vi "GeneralConfigMain.vi"(6 "NameSpace(Config)":string="Config", 8 "RIOfileName":string, 9 "Stop_Notifier":refnum<notifier>, 10 "IP_Notifier":refnum<notifier>, 11 "BasePath":path) -> ()   [LabVIEW 2016]
panel:
  in  "ViewCfgOnBot":bool
  in  "ULConfigtoRIO":bool
  in  "ConfigSaves":i32(listbox)=9
  in  "ConfigName":string
  in  "DeleteConfig":bool
  in  "LoadConfig":bool
  in  "SaveConfig":bool
  in  "Tab Control":enum32{"Page 1", "Page 2"}(tab)
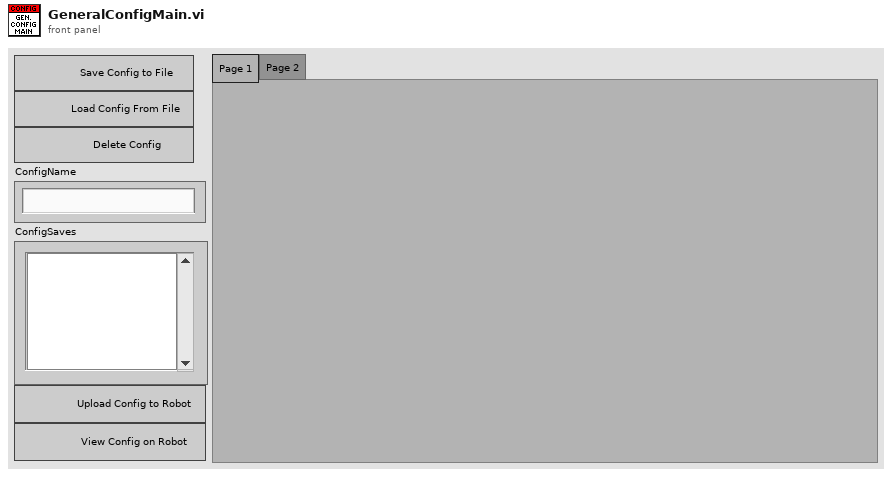
[diagram p1: front panel]
types:
  T1 = cluster{"ViewCfgOnBot":refnum<vi>, "ULConfigtoRIO":refnum<vi>, "ConfigSaves":refnum<vi>, "ConfigName":refnum<vi>, "DeleteConfig":refnum<vi>, "LoadConfig":refnum<vi>, "SaveConfig":refnum<vi>, "Stop_Notifier":refnum<notifier>, "IP_Notifier":refnum<notifier>, "appended path":path, "RIOfileName":string}
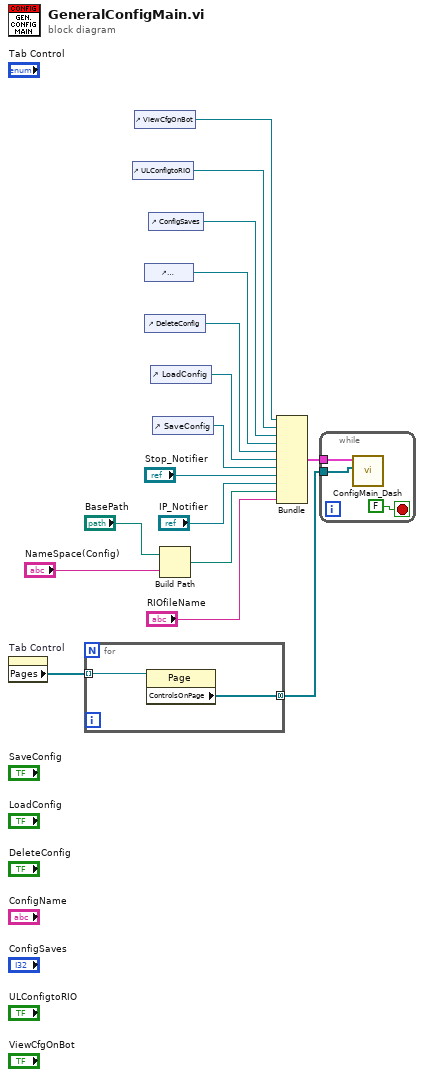
[diagram p0: block diagram]
diagram:
  n1 = property on="Tab Control" class="TabCtl (strict)"() -> ("Pages"=w16:refnum<vi>[])  [unwired: 2 in, 2 out]
  n2 = for {
    tunnel: w16 -> [w18] mode=indexing
    tunnel: [w17] -> w6 mode=concatenating
    n3 = property class="Page"(reference=w18) -> ("ControlsOnPage"=w17:refnum<vi>[])  [unwired: 1 in, 2 out]
  }
  n4 = control-ref of="ULConfigtoRIO"() -> (w14:refnum<vi>)
  n5 = control-ref of="ViewCfgOnBot"() -> (w15:refnum<vi>)
  n6 = control-ref of="ConfigName"() -> (w12:refnum<vi>)
  n7 = control-ref of="DeleteConfig"() -> (w11:refnum<vi>)
  n8 = control-ref of="ConfigSaves"() -> (w13:refnum<vi>)
  n9 = control-ref of="LoadConfig"() -> (w10:refnum<vi>)
  n10 = control-ref of="SaveConfig"() -> (w9:refnum<vi>)
  n11 = Build Path(base path="BasePath", name or relative path="NameSpace(Config)") -> (appended path=w1:path)
  n12 = Bundle("ViewCfgOnBot"=w15, "ULConfigtoRIO"=w14, "ConfigSaves"=w13, "ConfigName"=w12, "DeleteConfig"=w11, "LoadConfig"=w10, "SaveConfig"=w9, "Stop_Notifier"="Stop_Notifier", "IP_Notifier"="IP_Notifier", "appended path"=w1, "RIOfileName"="RIOfileName") -> (w5:T1)  [unwired: 1 in]
  n13 = while {
    tunnel: w6 -> [w21]
    tunnel: w5 -> [w20]
    stop <- FALSE stop-if-true
    n14 = call "ConfigMain_Dash.vi"("ControlsToSave"=w21, "ControlElements"=w20) -> ()  [unwired: 10 in]
  }
